vi "Poll Freezers.vi"(8 "error in (no error)":errorcluster, 11 "cRIO-CO2 in":refnum<class "cRIO-CO2.lvclass">) -> (0 "error out":errorcluster)   [LabVIEW 2015, in "cRIO-Carbondioxide.lvlib" / "cRIO-CO2.lvlib" / "cRIO-CO2.lvclass"]
uses:
  cRIO-CO2.lvclass
  <vilib>/ActorFramework/Actor/Actor.lvclass/Actor.ctl
  <vilib>/ActorFramework/Message Enqueuer/Message Enqueuer.lvclass/Message Enqueuer.ctl
  Freezers Enumerator.ctl
  cRIO-CO2 Messages/Launch Freezer Msg/Launch Freezer Msg.lvclass/Launch Freezer Msg.ctl
  <vilib>/ActorFramework/Message Enqueuer/Init from Existing Queue.vi
  <vilib>/ActorFramework/Message Enqueuer/Enqueue.vi
  <vilib>/ActorFramework/Message Priority Queue/Priority Enqueue.vi
  <vilib>/ActorFramework/Message Enqueuer/Message Enqueuer.lvclass
  cRIO-CO2 Messages/Launch Freezer Msg/Launch Freezer Msg.lvclass
  <vilib>/ActorFramework/Actor/Actor.lvclass
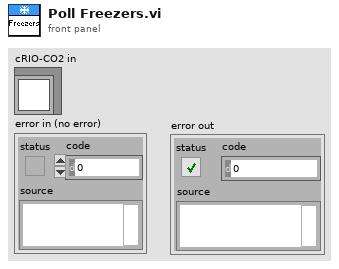
[diagram p1: front panel]
types:
  T1 = typedef "cRIO-Carbondioxide.lvlib/cRIO-CO2.lvlib/cRIO-CO2.lvclass/Freezers Enumerator.ctl" = enum16{"Undefined", "Syringe", "Cold Tank 1", "Cold Tank 2", "Cold Tank 3", "Cold Tank 4"}
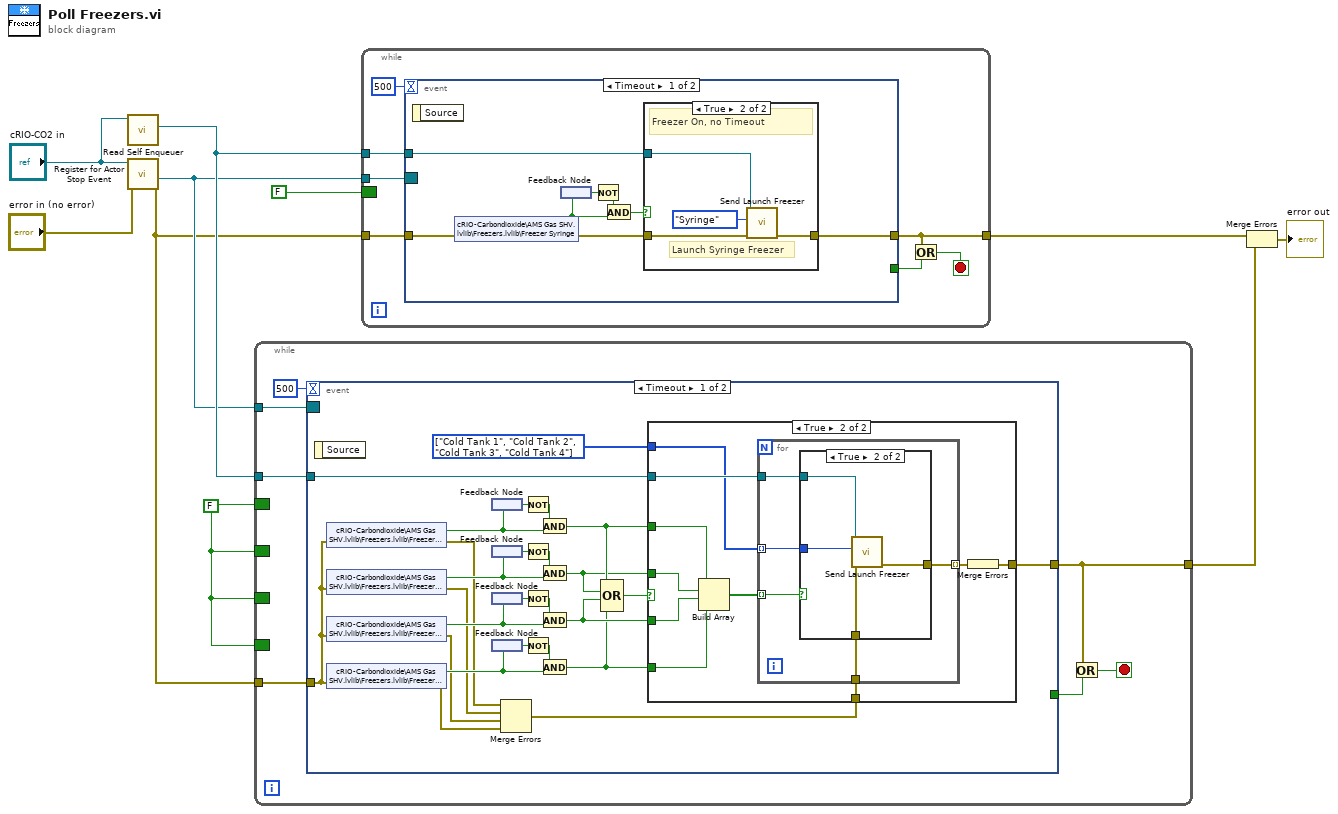
[diagram p0: block diagram]
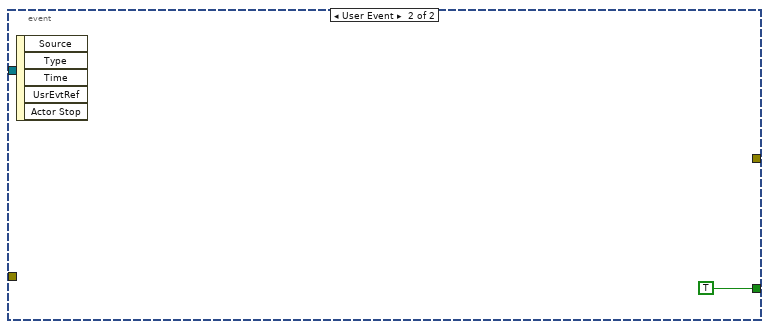
[diagram p4: hidden frame]
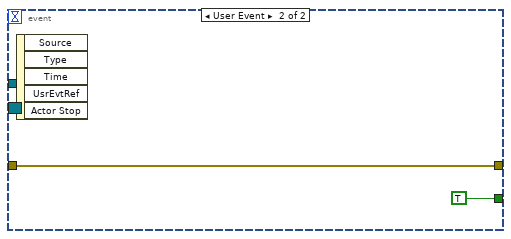
[diagram p6: hidden frame]
diagram:
  w5 = FALSE ("Boolean")
  n1 = call <vilib>:"Read Self Enqueuer.vi"("Actor"="cRIO-CO2 in") -> ("Self Enqueuer"=w7:refnum<class "Message Enqueuer.lvclass">)  [unwired: 10 in]
  n2 = call "Register for Actor Stop Event.vi"("error in (no error)"="error in (no error)", "cRIO-CO2 in"="cRIO-CO2 in") -> ("error out"=w4:errorcluster, "Event Registration Refnum"=w6:refnum<event-registration>)  [unwired: 7 in, 1 out]
  n3 = while {
    tunnel: w7 -> [w17]
    border: w5 -> [_]
    tunnel: w6 -> [w16]
    border: w5 -> [_]
    border: w5 -> [_]
    border: w5 -> [_]
    tunnel: w4 -> [w12]
    tunnel: [w11] -> w2
    stop <- w13 stop-if-true
    n4 = event shown="[0] Timeout" {
      selector: w16 -> [_ _]
      dyn-events: _ -> [_ _]
      timeout: 500 -> [_ _]
      tunnel: w17 -> [w34 _]
      tunnel: [_ TRUE] -> w14
      tunnel: [w19 _] -> w11
      tunnel: w12 -> [w18 _]
      event Timeout {
        w29 = T1[] [enum."Cold Tank 1", enum."Cold Tank 2", enum."Cold Tank 3", enum."Cold Tank 4"] items=["Undefined", "Syringe", "Cold Tank 1", "Cold Tank 2", "Cold Tank 3", "Cold Tank 4"]
        n5 = event-data() -> ()  [unwired: 1 in, 1 out]
        n6 = shared-variable "cRIO-Carbondioxide\\AMS Gas SHV.lvlib\\Freezers.lvlib\\Freezer Tank 1"(error in=w18) -> (w27:bool, error out=w24:errorcluster)
        n7 = shared-variable "cRIO-Carbondioxide\\AMS Gas SHV.lvlib\\Freezers.lvlib\\Freezer Tank 2"(error in=w18) -> (w28:bool, error out=w23:errorcluster)
        n8 = shared-variable "cRIO-Carbondioxide\\AMS Gas SHV.lvlib\\Freezers.lvlib\\Freezer Tank 3"(error in=w18) -> (w26:bool, error out=w22:errorcluster)
        n9 = shared-variable "cRIO-Carbondioxide\\AMS Gas SHV.lvlib\\Freezers.lvlib\\Freezer Tank 4"(error in=w18) -> (w25:bool, error out=w21:errorcluster)
        n10 = feedback #1() -> (w43:bool)
        n11 = feedback-in #1(w27) -> ()
        n12 = feedback #2() -> (w40:bool)
        n13 = feedback-in #2(w28) -> ()
        n14 = feedback #3() -> (w39:bool)
        n15 = feedback-in #3(w26) -> ()
        n16 = feedback #4() -> (w36:bool)
        n17 = feedback-in #4(w25) -> ()
        n18 = Merge Errors(w24, w23, w22, w21) -> (w20:errorcluster)
        n19 = Not(x=w43) -> (.not. x?=w42:bool)
        n20 = Not(x=w40) -> (.not. x?=w41:bool)
        n21 = Not(x=w39) -> (.not. x?=w38:bool)
        n22 = Not(x=w36) -> (.not. x?=w37:bool)
        n23 = And(x=w42, y=w27) -> (x .and. y?=w33:bool)
        n24 = And(x=w41, y=w28) -> (x .and. y?=w32:bool)
        n25 = And(x=w38, y=w26) -> (x .and. y?=w31:bool)
        n26 = And(x=w37, y=w25) -> (x .and. y?=w30:bool)
        n27 = Compound Arithmetic op=OR(w33, w32, w31, w30) -> (w35:bool)
        n28 = case shown="True" w35 {
          tunnel: w34 -> [_ w49]
          tunnel: w33 -> [_ w54]
          tunnel: w32 -> [_ w53]
          tunnel: w31 -> [_ w52]
          tunnel: w30 -> [_ w51]
          tunnel: w29 -> [_ w48]
          tunnel: w20 -> [w44 w47]
          tunnel: [w44 w45] -> w19
          frame False {
          }
          frame True {
            n29 = Build Array(w54, w53, w52, w51) -> (w50:bool[])
            n30 = for {
              tunnel: w50 -> [w59] mode=indexing
              tunnel: w49 -> [w57]
              tunnel: w48 -> [w58] mode=indexing
              tunnel: w47 -> [w56]
              tunnel: [w55] -> w46 mode=indexing
              n31 = case shown="True" w59 {
                tunnel: w58 -> [_ w63]
                tunnel: w57 -> [_ w64]
                tunnel: w56 -> [w60 w62]
                tunnel: [w60 w61] -> w55
                frame False {
                }
                frame True {
                  n32 = call "Send Launch Freezer.vi"("error in (no error)"=w62, "Freezer"=w63, "Message Enqueuer"=w64) -> ("error out"=w61:errorcluster)  [unwired: 7 in, 1 out]
                }
              }
            }
            n33 = Merge Errors(w46) -> (w45:errorcluster)
          }
        }
      }
      event User Event {
        n34 = event-data() -> ()  [unwired: 1 in, 5 out]
      }
    }
    n35 = Or(x=w11, y=w14) -> (x .or. y?=w13:bool)
  }
  n36 = while {
    tunnel: w7 -> [w72]
    border: FALSE ("Boolean") -> [_]
    tunnel: w6 -> [w71]
    tunnel: w4 -> [w70]
    tunnel: [w66] -> w3
    stop <- w67 stop-if-true
    n37 = event shown="[0] Timeout" {
      selector: w71 -> [_ _]
      dyn-events: _ -> [_ _]
      timeout: 500 -> [_ _]
      tunnel: [w80 w86] -> w66
      tunnel: w72 -> [w78 _]
      tunnel: w70 -> [w73 w86]
      tunnel: [_ TRUE] -> w68
      event Timeout {
        n38 = event-data() -> ()  [unwired: 1 in, 1 out]
        n39 = shared-variable "cRIO-Carbondioxide\\AMS Gas SHV.lvlib\\Freezers.lvlib\\Freezer Syringe"(error in=w73) -> (w76:bool, error out=w79:errorcluster)
        n40 = feedback #5() -> (w75:bool)
        n41 = feedback-in #5(w76) -> ()
        n42 = Not(x=w75) -> (.not. x?=w74:bool)
        n43 = And(x=w74, y=w76) -> (x .and. y?=w77:bool)
        n44 = case shown="True" w77 {
          tunnel: w78 -> [_ w83]
          tunnel: [w81 w84] -> w80
          tunnel: w79 -> [w81 w85]
          frame False {
          }
          frame True {
            # "Launch Syringe Freezer"
            # "Freezer On, no Timeout"
            n45 = call "Send Launch Freezer.vi"("error in (no error)"=w85, "Freezer"=Freezers_Enumerator."Syringe", "Message Enqueuer"=w83) -> ("error out"=w84:errorcluster)  [unwired: 7 in, 1 out]
          }
        }
      }
      event User Event {
        n46 = event-data() -> ()  [unwired: 1 in, 5 out]
      }
    }
    n47 = Or(x=w66, y=w68) -> (x .or. y?=w67:bool)
  }
  n48 = Merge Errors(w3, w2) -> (→"error out":errorcluster)
